vi "Begin by Value.vi"(8 "Error In":errorcluster, 10 "Msgpack Data":u8[](array[numeric]), 11 "Reader In":refnum<class "Reader.lvclass">) -> (0 "Error Out":errorcluster, 3 "Reader Out":refnum<class "Reader.lvclass">)   [LabVIEW 2019, in "LabPack.lvlib" / "Reader.lvclass"]
uses:
  Reader.lvclass
  Reader.lvclass/Reader.ctl
  Public/Status/Read Status.vi
  Public/Status/Read Status Message.vi
  Public/Status/Read Is Error.vi
  Utility/Status Code.vi
  <vilib>/Utility/error.llb/Error Cluster From Error Code.vi
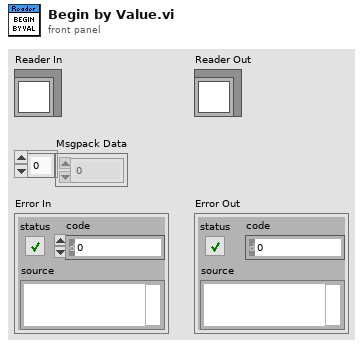
[diagram p1: front panel]
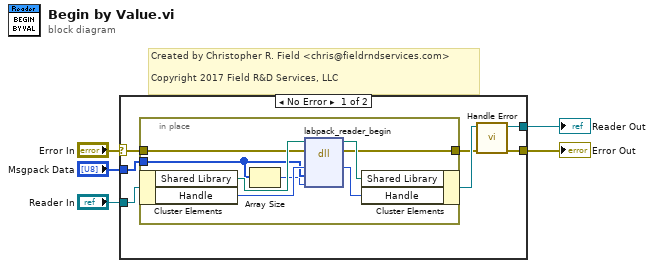
[diagram p0: block diagram]
diagram:
  # "Created by Christopher R. Field <chris@fieldrndservices.com>\n\nCopyright 2017 Field R&D Services, LLC"
  n1 = case shown="No Error" "Error In" {
    selector: "Error In" -> [w11 w22]
    tunnel: "Reader In" -> [w12 w21]
    tunnel: [w6 w22] -> w3
    tunnel: [w8 w21] -> w2
    tunnel: "Msgpack Data" -> [w9 _]
    frame No Error {
      n2 = in-place {
        in-place-border: w11 -> [w16]
        in-place-border: [w15] -> w7
        in-place-border: w9 -> [w14]
        n3 = in-place-cluster #1(w12) -> ("Shared Library"=w20:path, "Handle"=w18:u64)
        n4 = Array Size(array=w14) -> (size(s)=w13:i32)
        n5 = dll-call lib="D:/Users/cfield/Code/MessagePack/LabPack/LabVIEW/trunk/src/LabPack/Private/labpack-x64.dll" fn="labpack_reader_begin"(path in=w20, error in=w16, "reader"=w18, "data"=w14, "count"=w13) -> (path out=w19:path, error out=w15:errorcluster, "reader"=w17:u64)  [unwired: 4 in]
        n6 = in-place-cluster #1("Shared Library"=w19, "Handle"=w17) -> (w10:refnum<class "Reader.lvclass">)
      }
      n7 = call "Handle Error.vi"("Error In"=w7, "Reader In"=w10) -> ("Error Out"=w6:errorcluster, "Reader Out"=w8:refnum<class "Reader.lvclass">)  [unwired: 8 in]
    }
    frame Error {
    }
  }
  "Error Out" <- w3
  "Reader Out" <- w2
